vi "Test_QueueTimer.vi"() -> (2 "Tests":cluster{"Test":string, "Passed":bool}[](array[cluster]), 3 "All Passed":bool)   [LabVIEW 2021]
uses:
  src/QueueTimer/QueueTimer.lvlib
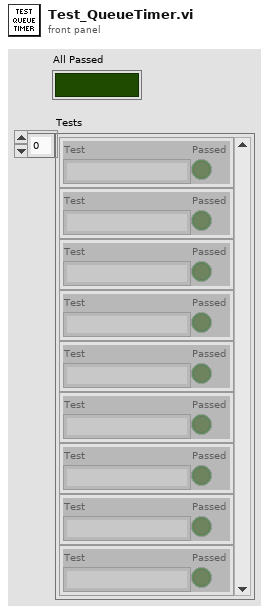
[diagram p1: front panel]
types:
  T1 = cluster{"Queue":refnum<queue>, "Messages":string[]}[]
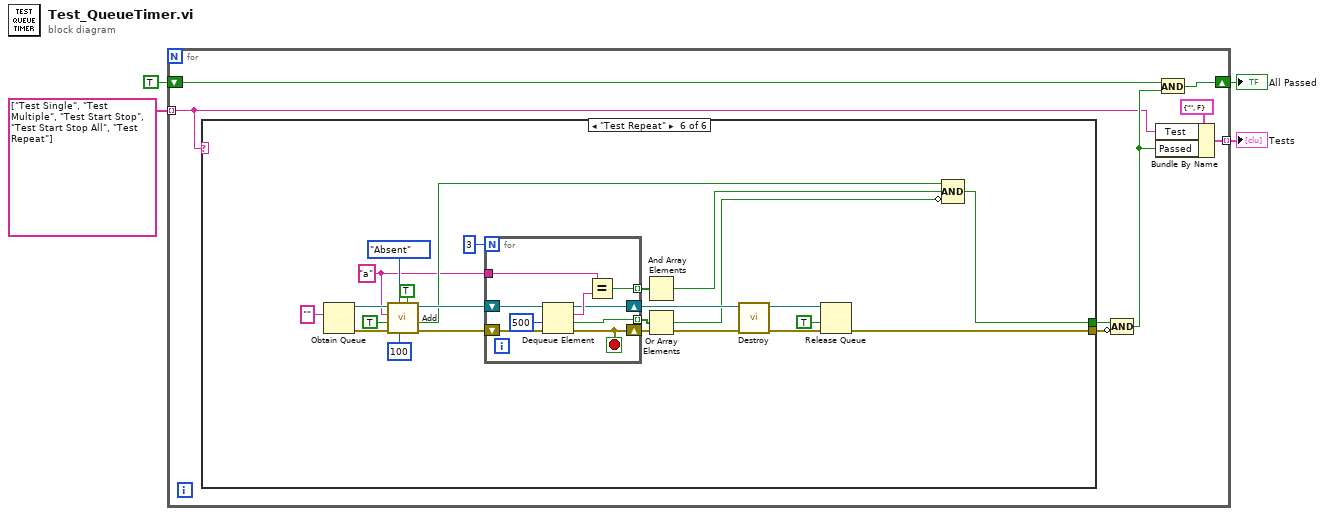
[diagram p0: block diagram]
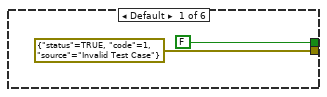
[diagram p2: hidden frame]
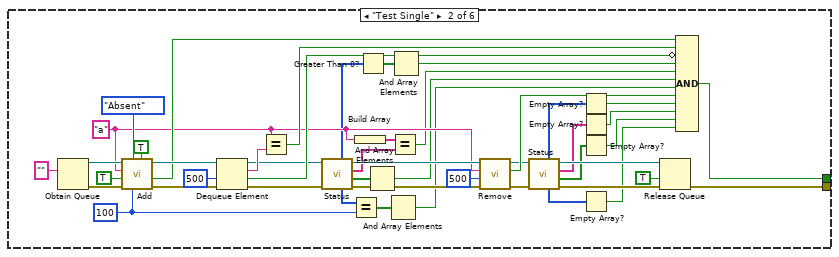
[diagram p3: hidden frame]
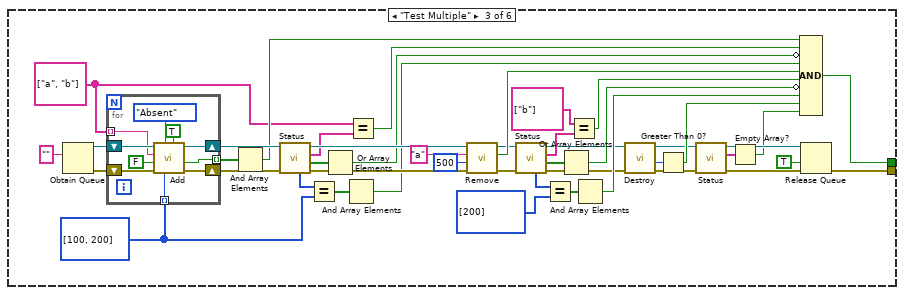
[diagram p4: hidden frame]
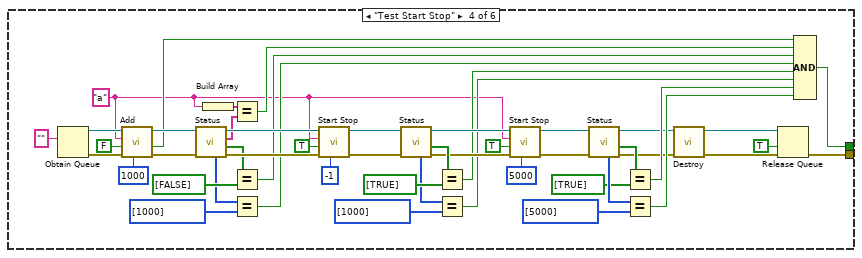
[diagram p5: hidden frame]
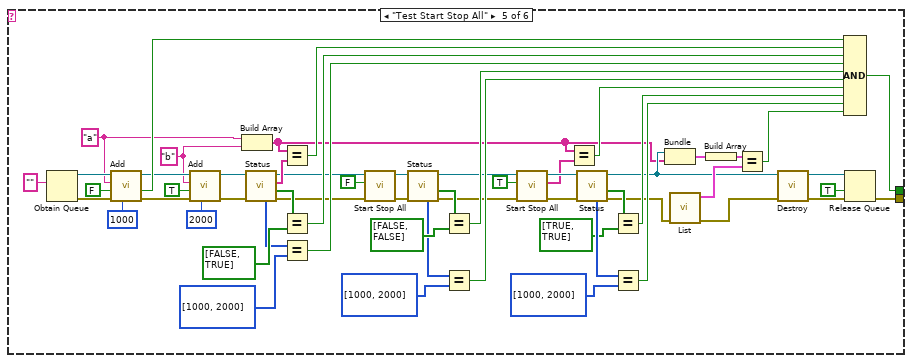
[diagram p6: hidden frame]
diagram:
  n1 = for {
    tunnel: string[] ["Test Single", "Test Multiple", "Test Start Stop", "Test Start Stop All", "Test Repeat"] -> [w5] mode=indexing
    shift-right: [w10] -> w2
    shift-left: TRUE -> [w11]
    tunnel: [w9] -> w1 mode=indexing
    n2 = case shown="\"Test Repeat\"" w5 {
      tunnel: [FALSE w45 w99 w159 w218 w234] -> w8
      tunnel: [errorcluster {"status"=TRUE, "code"=1, "source"="Invalid Test Case"} ("error in (no error)") w46 w100 w160 w219 w235] -> w6
      frame Default {
      }
      frame "Test Single" {
        w29 = 100 ("ms Delay (1000)")
        w39 = "a" ("Timer Message")
        n3 = Obtain Queue(element data type="") -> (queue out=w60:refnum<queue>, error out=w59:errorcluster)  [unwired: 4 in, 1 out]
        n4 = call "Add.vi"("Create if not Found? (T)"=TRUE, "ms Delay (1000)"=w29, "Method (Absent)"=enum8{"Back", "Front", "Lossy", "Absent"}."Absent", "error in (no error)"=w59, "Start? (T)"=TRUE, "Timer Message"=w39, "Queue in"=w60) -> ("error out"=w54:errorcluster, "Created New?"=w52:bool, "Queue out"=w55:refnum<queue>)  [unwired: 2 in]
        n5 = Dequeue Element(queue=w55, timeout in ms (-1)=500, error in (no error)=w54) -> (queue out=w42:refnum<queue>, element=w49:string, timed out?=w47:bool, error out=w44:errorcluster)
        n6 = Equal?(x=w39, y=w49) -> (x = y?=w48:bool)
        n7 = call "Status.vi"("error in (no error)"=w44, "Queue in"=w42) -> ("error out"=w43:errorcluster, "Running"=w32:bool[], "Timer Messages"=w40:string[], "Queue out"=w41:refnum<queue>, "Delay (ms)"=w30:i32[], "Last Ticks (ms)"=w35:u32[])  [unwired: 4 in]
        n8 = Equal?(x=w30, y=w29) -> (x = y?=w28:bool[])
        n9 = Build Array(w39) -> (w38:string[])
        n10 = Greater Than 0?(x=w35) -> (x > 0?=w34:bool[])
        n11 = And Array Elements(Boolean array=w32) -> (logical AND=w31:bool)
        n12 = And Array Elements(Boolean array=w28) -> (logical AND=w27:bool)
        n13 = Equal?(x=w38, y=w40) -> (x = y?=w36:bool)
        n14 = And Array Elements(Boolean array=w34) -> (logical AND=w33:bool)
        n15 = call "Remove.vi"("error in (no error)"=w43, "ms Timeout (500)"=u32 500 ("ms Timeout (2000)"), "Timer Message"=w39, "Queue in"=w41) -> ("error out"=w26:errorcluster, "Found?"=w37:bool, "Queue out"=w25:refnum<queue>)  [unwired: 5 in]
        n16 = call "Status.vi"("error in (no error)"=w26, "Queue in"=w25) -> ("error out"=w24:errorcluster, "Running"=w18:bool[], "Timer Messages"=w20:string[], "Queue out"=w23:refnum<queue>, "Delay (ms)"=w16:i32[], "Last Ticks (ms)"=w22:u32[])  [unwired: 4 in]
        n17 = Empty Array?(array=w22) -> (empty?=w21:bool)
        n18 = Empty Array?(array=w20) -> (empty?=w19:bool)
        n19 = Empty Array?(array=w18) -> (empty?=w17:bool)
        n20 = Empty Array?(array=w16) -> (empty?=w15:bool)
        n21 = Release Queue(queue=w23, force destroy? (F)=TRUE, error in (no error)=w24) -> (error out=w46:errorcluster)  [unwired: 2 out]
        n22 = Compound Arithmetic op=AND(w52, w48, invert w47, w33, w36, w31, w27, w37, w21, w19, w17, w15) -> (w45:bool)
      }
      frame "Test Multiple" {
        w89 = i32[] [100, 200]
        w85 = string[] ["a", "b"]
        n23 = Obtain Queue(element data type="") -> (queue out=w105:refnum<queue>, error out=w104:errorcluster)  [unwired: 4 in, 1 out]
        n24 = for {
          tunnel: [w109] -> w103 mode=indexing
          shift-right: [w111] -> w87
          shift-left: w105 -> [w116]
          shift-right: [w110] -> w88
          shift-left: w104 -> [w115]
          tunnel: w85 -> [w108] mode=indexing
          tunnel: w89 -> [w107] mode=indexing
          n25 = call "Add.vi"("Create if not Found? (T)"=TRUE, "ms Delay (1000)"=w107, "Method (Absent)"=enum8{"Back", "Front", "Lossy", "Absent"}."Absent", "error in (no error)"=w115, "Start? (T)"=FALSE, "Timer Message"=w108, "Queue in"=w116) -> ("error out"=w110:errorcluster, "Created New?"=w109:bool, "Queue out"=w111:refnum<queue>)  [unwired: 2 in]
        }
        n26 = And Array Elements(Boolean array=w103) -> (logical AND=w86:bool)
        n27 = call "Status.vi"("error in (no error)"=w88, "Queue in"=w87) -> ("error out"=w98:errorcluster, "Running"=w93:bool[], "Timer Messages"=w96:string[], "Queue out"=w97:refnum<queue>, "Delay (ms)"=w92:i32[])  [unwired: 4 in, 1 out]
        n28 = Equal?(x=w92, y=w89) -> (x = y?=w91:bool[])
        n29 = Or Array Elements(Boolean array=w93) -> (logical OR=w84:bool)
        n30 = And Array Elements(Boolean array=w91) -> (logical AND=w90:bool)
        n31 = Equal?(x=w85, y=w96) -> (x = y?=w94:bool)
        n32 = call "Remove.vi"("error in (no error)"=w98, "ms Timeout (500)"=u32 500 ("ms Timeout (2000)"), "Timer Message"="a", "Queue in"=w97) -> ("error out"=w78:errorcluster, "Found?"=w95:bool, "Queue out"=w77:refnum<queue>)  [unwired: 5 in]
        n33 = call "Status.vi"("error in (no error)"=w78, "Queue in"=w77) -> ("error out"=w70:errorcluster, "Running"=w80:bool[], "Timer Messages"=w79:string[], "Queue out"=w71:refnum<queue>, "Delay (ms)"=w81:i32[])  [unwired: 4 in, 1 out]
        n34 = Equal?(x=w81, y=i32[] [200]) -> (x = y?=w82:bool[])
        n35 = Or Array Elements(Boolean array=w80) -> (logical OR=w73:bool)
        n36 = Equal?(x=string[] ["b"], y=w79) -> (x = y?=w74:bool)
        n37 = And Array Elements(Boolean array=w82) -> (logical AND=w72:bool)
        n38 = call "Destroy.vi"("error in (no error)"=w70, "Queue in"=w71) -> ("error out"=w67:errorcluster, "ms Elapsed"=w69:u32, "Queue out"=w66:refnum<queue>)  [unwired: 7 in]
        n39 = Greater Than 0?(x=w69) -> (x > 0?=w68:bool)
        n40 = call "Status.vi"("error in (no error)"=w67, "Queue in"=w66) -> ("error out"=w65:errorcluster, "Timer Messages"=w63:string[], "Queue out"=w64:refnum<queue>)  [unwired: 4 in, 3 out]
        n41 = Empty Array?(array=w63) -> (empty?=w62:bool)
        n42 = Compound Arithmetic op=AND(w86, w94, invert w84, w90, w95, w74, invert w73, w72, w68, w62) -> (w99:bool)
        n43 = Release Queue(queue=w64, force destroy? (F)=TRUE, error in (no error)=w65) -> (error out=w100:errorcluster)  [unwired: 2 out]
      }
      frame "Test Start Stop" {
        w117 = "a" ("Timer Message")
        n44 = Obtain Queue(element data type="") -> (queue out=w164:refnum<queue>, error out=w163:errorcluster)  [unwired: 4 in, 1 out]
        n45 = call "Add.vi"("ms Delay (1000)"=1000, "error in (no error)"=w163, "Start? (T)"=FALSE, "Timer Message"=w117, "Queue in"=w164) -> ("error out"=w156:errorcluster, "Created New?"=w155:bool, "Queue out"=w157:refnum<queue>)  [unwired: 4 in]
        n46 = call "Status.vi"("error in (no error)"=w156, "Queue in"=w157) -> ("error out"=w153:errorcluster, "Running"=w151:bool[], "Timer Messages"=w124:string[], "Queue out"=w154:refnum<queue>, "Delay (ms)"=w138:i32[])  [unwired: 4 in, 1 out]
        n47 = Build Array(w117) -> (w123:string[])
        n48 = Equal?(x=w123, y=w124) -> (x = y?=w122:bool)
        n49 = Equal?(x=w151, y=bool[] [FALSE]) -> (x = y?=w149:bool)
        n50 = Equal?(x=w138, y=i32[] [1000]) -> (x = y?=w134:bool)
        n51 = call "Start Stop.vi"("ms Delay (-1=No change)"=-1, "error in (no error)"=w153, "Start? (T)"=TRUE, "Timer Message"=w117, "Queue in"=w154) -> ("error out"=w141:errorcluster, "Queue out"=w140:refnum<queue>)  [unwired: 5 in]
        n52 = call "Status.vi"("error in (no error)"=w141, "Queue in"=w140) -> ("error out"=w143:errorcluster, "Running"=w145:bool[], "Queue out"=w142:refnum<queue>, "Delay (ms)"=w135:i32[])  [unwired: 4 in, 2 out]
        n53 = Equal?(x=w145, y=bool[] [TRUE]) -> (x = y?=w139:bool)
        n54 = Equal?(x=w135, y=i32[] [1000]) -> (x = y?=w133:bool)
        n55 = call "Start Stop.vi"("ms Delay (-1=No change)"=5000, "error in (no error)"=w143, "Start? (T)"=TRUE, "Timer Message"=w117, "Queue in"=w142) -> ("error out"=w128:errorcluster, "Queue out"=w127:refnum<queue>)  [unwired: 5 in]
        n56 = call "Status.vi"("error in (no error)"=w128, "Queue in"=w127) -> ("error out"=w121:errorcluster, "Running"=w130:bool[], "Queue out"=w119:refnum<queue>, "Delay (ms)"=w132:i32[])  [unwired: 4 in, 2 out]
        n57 = Equal?(x=w130, y=bool[] [TRUE]) -> (x = y?=w126:bool)
        n58 = Equal?(x=w132, y=i32[] [5000]) -> (x = y?=w125:bool)
        n59 = call "Destroy.vi"("error in (no error)"=w121, "Queue in"=w119) -> ("error out"=w120:errorcluster, "Queue out"=w118:refnum<queue>)  [unwired: 7 in, 1 out]
        n60 = Release Queue(queue=w118, force destroy? (F)=TRUE, error in (no error)=w120) -> (error out=w160:errorcluster)  [unwired: 2 out]
        n61 = Compound Arithmetic op=AND(w155, w122, w149, w134, w139, w133, w126, w125) -> (w159:bool)
      }
      frame "Test Start Stop All" {
        w192 = "b" ("Timer Message")
        w199 = "a" ("Timer Message")
        n62 = Obtain Queue(element data type="") -> (queue out=w223:refnum<queue>, error out=w222:errorcluster)  [unwired: 4 in, 1 out]
        n63 = call "Add.vi"("ms Delay (1000)"=1000, "error in (no error)"=w222, "Start? (T)"=FALSE, "Timer Message"=w199, "Queue in"=w223) -> ("error out"=w195:errorcluster, "Created New?"=w216:bool, "Queue out"=w196:refnum<queue>)  [unwired: 4 in]
        n64 = call "Add.vi"("ms Delay (1000)"=2000, "error in (no error)"=w195, "Start? (T)"=TRUE, "Timer Message"=w192, "Queue in"=w196) -> ("error out"=w193:errorcluster, "Queue out"=w194:refnum<queue>)  [unwired: 4 in, 1 out]
        n65 = Build Array(w199, w192) -> (w169:string[])
        n66 = call "Status.vi"("error in (no error)"=w193, "Queue in"=w194) -> ("error out"=w191:errorcluster, "Running"=w215:bool[], "Timer Messages"=w203:string[], "Queue out"=w189:refnum<queue>, "Delay (ms)"=w209:i32[])  [unwired: 4 in, 1 out]
        n67 = Equal?(x=w169, y=w203) -> (x = y?=w202:bool)
        n68 = Equal?(x=w215, y=bool[] [FALSE, TRUE]) -> (x = y?=w213:bool)
        n69 = Equal?(x=w209, y=i32[] [1000, 2000]) -> (x = y?=w205:bool)
        n70 = call "Start Stop All.vi"("error in (no error)"=w191, "Start? (T)"=FALSE, "Queue in"=w189) -> ("error out"=w190:errorcluster, "Queue out"=w188:refnum<queue>)  [unwired: 6 in, 1 out]
        n71 = call "Status.vi"("error in (no error)"=w190, "Queue in"=w188) -> ("error out"=w178:errorcluster, "Running"=w211:bool[], "Queue out"=w179:refnum<queue>, "Delay (ms)"=w206:i32[])  [unwired: 4 in, 2 out]
        n72 = Equal?(x=w211, y=bool[] [FALSE, FALSE]) -> (x = y?=w210:bool)
        n73 = Equal?(x=w206, y=i32[] [1000, 2000]) -> (x = y?=w204:bool)
        n74 = call "Start Stop All.vi"("error in (no error)"=w178, "Start? (T)"=TRUE, "Queue in"=w179) -> ("error out"=w184:errorcluster, "Timer Messages"=w175:string[], "Queue out"=w185:refnum<queue>)  [unwired: 6 in]
        n75 = Equal?(x=w169, y=w175) -> (x = y?=w174:bool)
        n76 = call "Status.vi"("error in (no error)"=w184, "Queue in"=w185) -> ("error out"=w173:errorcluster, "Running"=w181:bool[], "Queue out"=w170:refnum<queue>, "Delay (ms)"=w183:i32[])  [unwired: 4 in, 2 out]
        n77 = Equal?(x=w181, y=bool[] [TRUE, TRUE]) -> (x = y?=w177:bool)
        n78 = Equal?(x=w183, y=i32[] [1000, 2000]) -> (x = y?=w176:bool)
        n79 = Bundle("Queue out"=w170, w169) -> (w168:cluster{"Queue out":refnum<queue>, string[]})  [unwired: 1 in]
        n80 = call "List.vi"("error in (no error)"=w173) -> ("error out"=w172:errorcluster, "All Timers"=w171:T1)  [unwired: 9 in]
        n81 = Build Array(w168) -> (w167:cluster{"Queue out":refnum<queue>, string[]}[])
        n82 = Equal?(x=w167, y=w171) -> (x = y?=w166:bool)
        n83 = call "Destroy.vi"("error in (no error)"=w172, "Queue in"=w170) -> ("error out"=w201:errorcluster, "Queue out"=w200:refnum<queue>)  [unwired: 7 in, 1 out]
        n84 = Compound Arithmetic op=AND(w216, w202, w213, w205, w210, w204, w174, w177, w176, w166) -> (w218:bool)
        n85 = Release Queue(queue=w200, force destroy? (F)=TRUE, error in (no error)=w201) -> (error out=w219:errorcluster)  [unwired: 2 out]
      }
      frame "Test Repeat" {
        w233 = "a" ("Timer Message")
        n86 = Obtain Queue(element data type="") -> (queue out=w246:refnum<queue>, error out=w245:errorcluster)  [unwired: 4 in, 1 out]
        n87 = call "Add.vi"("Create if not Found? (T)"=TRUE, "ms Delay (1000)"=100, "Method (Absent)"=enum8{"Back", "Front", "Lossy", "Absent"}."Absent", "error in (no error)"=w245, "Start? (T)"=TRUE, "Timer Message"=w233, "Queue in"=w246) -> ("error out"=w240:errorcluster, "Created New?"=w239:bool, "Queue out"=w241:refnum<queue>)  [unwired: 2 in]
        n88 = for {
          N: 3 -> [_]
          tunnel: [w252] -> w237 mode=indexing
          tunnel: [w251] -> w236 mode=indexing
          tunnel: w233 -> [w250]
          shift-right: [w249] -> w228
          shift-left: w241 -> [w256]
          shift-right: [w248] -> w229
          shift-left: w240 -> [w255]
          stop <- w248 stop-if-true
          n89 = Dequeue Element(queue=w256, timeout in ms (-1)=500, error in (no error)=w255) -> (queue out=w249:refnum<queue>, element=w253:string, timed out?=w251:bool, error out=w248:errorcluster)
          n90 = Equal?(x=w250, y=w253) -> (x = y?=w252:bool)
        }
        n91 = And Array Elements(Boolean array=w237) -> (logical AND=w225:bool)
        n92 = Or Array Elements(Boolean array=w236) -> (logical OR=w226:bool)
        n93 = call "Destroy.vi"("error in (no error)"=w229, "Queue in"=w228) -> ("error out"=w230:errorcluster, "Queue out"=w231:refnum<queue>)  [unwired: 7 in, 1 out]
        n94 = Release Queue(queue=w231, force destroy? (F)=TRUE, error in (no error)=w230) -> (error out=w235:errorcluster)  [unwired: 2 out]
        n95 = Compound Arithmetic op=AND(w239, w225, invert w226) -> (w234:bool)
      }
    }
    n96 = Compound Arithmetic op=AND(w8, invert w6) -> (w7:bool)
    n97 = Bundle By Name(cluster=cluster{"Test":string, "Passed":bool} {"Test"="", "Passed"=FALSE} ("Cluster"), "Test"=w5, "Passed"=w7) -> (w9:cluster{"Test":string, "Passed":bool})
    n98 = And(x=w11, y=w7) -> (x .and. y?=w10:bool)
  }
  "All Passed" <- w2
  "Tests" <- w1
